vi "Get Direction.vi"(8 "error in":errorcluster, 11 "message or subaddress":T2 format="%.0x") -> (0 "error out":errorcluster, 2 "direction":T1, 3 "message or subaddress out":T2 format="%.0x", 4 "found?":bool)   [LabVIEW 2020, in "AIM MIL-STD-1553 Scripting.lvlib"]
doc: "Returns the configured <b>direction</b> for the <b>message or subaddress</b>. If the specified <b>message or subaddress</b> is not found, <b>found?</b> returns a False."
uses:
  AIM MIL-STD-1553 Scripting.lvlib
  <vilib>/NI VeriStand/Custom Device API/Custom Device Item Ref.ctl
  Shared/Direction.ctl
  Constants.vi
  <vilib>/NI VeriStand/Custom Device API/Get Item Property (U16).vi
  <vilib>/NI VeriStand/Custom Device API/Custom Device API.lvlib
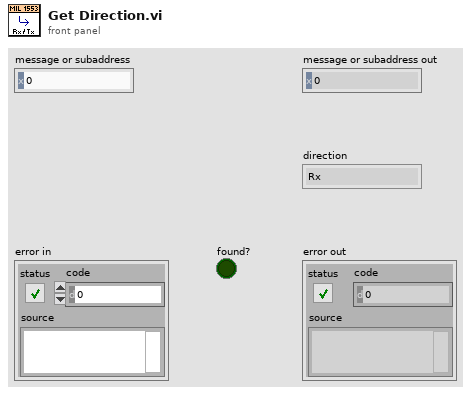
[diagram p1: front panel]
types:
  T1 = typedef "Direction.ctl" = enum16{"Rx", "Tx"}
  T2 = typedef "Custom Device API.lvlib/Custom Device Item Ref.ctl" = u64
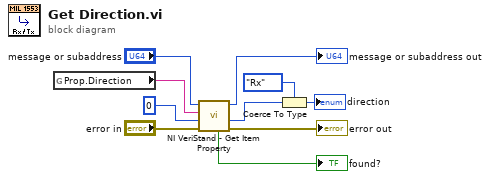
[diagram p0: block diagram]
diagram:
  n1 = global read "Constants.vi" "Prop.Direction"() -> (w6:string)
  n2 = call-poly <vilib>:"NI VeriStand - Get Item Property.vi"("error in (no error)"="error in", "Default Value"=u16 0 ("number of words"), "Property Name"=w6, "Item Ref in"="message or subaddress") -> ("error out"=→"error out":errorcluster, "Value"=w4:u16, "Item Ref out"=→"message or subaddress out":T2, "Found?"=→"found?":bool)  [unwired: 4 in]
  n3 = Coerce To Type(0:w4, 1:Direction."Rx" ("direction")) -> (2:→"direction":T1)
